vi "get async stop notifier.vi"(8 "error in":errorcluster {"code" format="Error %.0f"}, 11 "NATS Client in":refnum<class "NATS Client.lvclass">) -> (0 "error out":errorcluster {"code" format="Error %.0f"}, 2 "async stop notifier":refnum<notifier>, 3 "NATS Client out":refnum<class "NATS Client.lvclass">)   [LabVIEW 2024, in "NATS Client.lvlib" / "NATS Client.lvclass"]
uses:
  NATS Client.lvclass
  NATS Client.lvclass/NATS Client.ctl
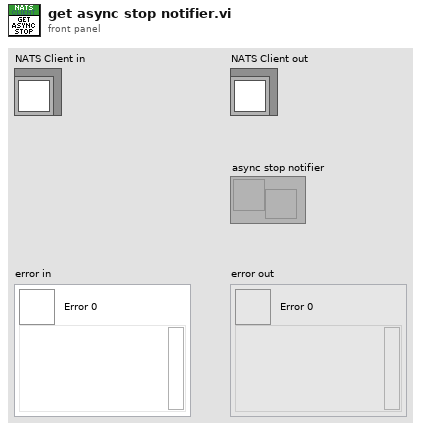
[diagram p1: front panel]
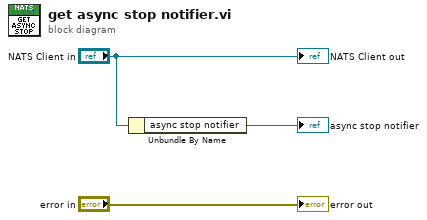
[diagram p0: block diagram]
diagram:
  n1 = Unbundle By Name("NATS Client in") -> ("async stop notifier"=→"async stop notifier":refnum<notifier>)
  "error out" <- "error in"
  "NATS Client out" <- "NATS Client in"
